vi "Cloud2.vi"() -> ()   [LabVIEW 2017]
uses:
  <vilib>/addons/_JKI.lib/REST Client/classes/REST Client/HTTP Header.ctl
  <vilib>/addons/_JKI.lib/REST Client/classes/REST Client/REST Client.lvclass
panel:
  out "error out 3":errorcluster
  out "error out 2":errorcluster
  out "F-format string":string
  in  "stop":bool
  out "Response body":string
  out "error out":errorcluster
  in  "Default Headers ([JSON])":T1[](array[typedef])=[{"header"="Content-Type", "value"="application/json"}]
  in  "error in (no error)":errorcluster
  in  "Authentication":cluster{"Username":string, "Password":string}
  in  "Base URL":string
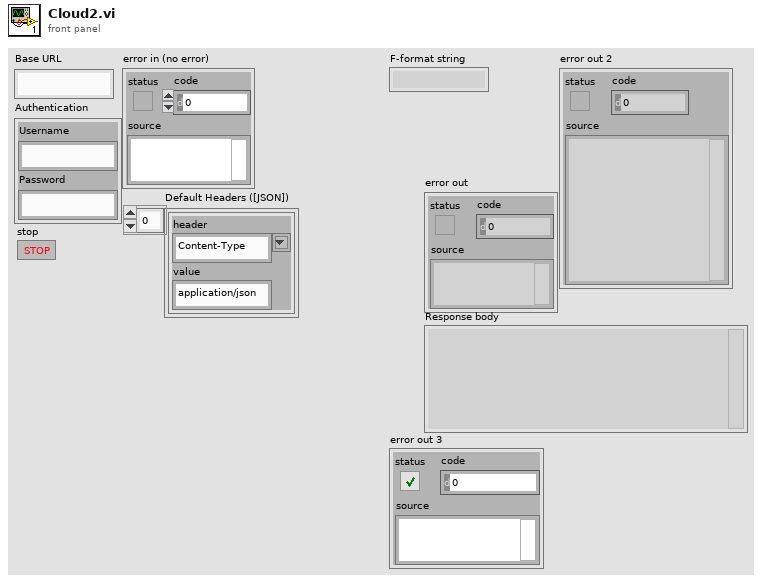
[diagram p1: front panel]
types:
  T1 = typedef "REST Client.lvlib/REST Client.lvclass/HTTP Header.ctl" = cluster{"header":string, "value":string}
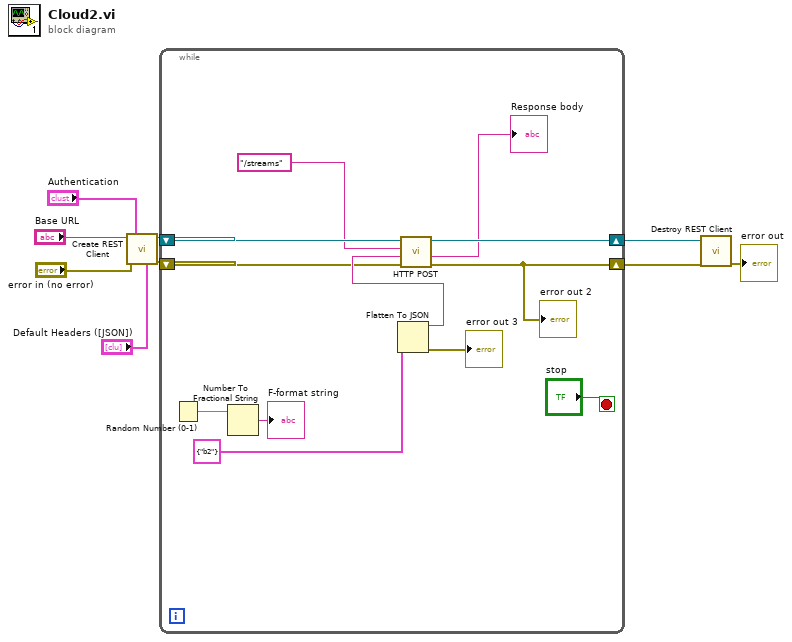
[diagram p0: block diagram]
diagram:
  n1 = call <vilib>:"Create REST Client.vi"("Default Headers ([JSON])"="Default Headers ([JSON])", "error in (no error)"="error in (no error)", "Authentication"="Authentication", "Base URL"="Base URL") -> ("error out"=w3:errorcluster, "REST Client out"=w9:refnum<class "REST Client.lvclass">)  [unwired: 6 in]
  n2 = while {
    shift-right: [w20] -> w8
    shift-left: w9 -> [w21]
    shift-right: [w11] -> w2
    shift-left: w3 -> [w14]
    stop <- "stop" stop-if-true
    n3 = Random Number (0-1)() -> (number: 0 to 1=w16:dbl)
    n4 = Number To Fractional String(number=w16) -> (F-format string=→"F-format string":string)  [unwired: 3 in]
    n5 = Flatten To JSON(anything=cluster{string} {"b2"}) -> (JSON string=w15:string, 11:→"error out 3":errorcluster)  [unwired: 2 in]
    n6 = call-dynamic "HTTP POST.vi"("error in (no error)"=w14, "Request body"=w15, "Path"="/streams", "REST Client in"=w21) -> ("error out"=w11:errorcluster, "Response body"=→"Response body":string, "REST Client out"=w20:refnum<class "REST Client.lvclass">)  [unwired: 2 in, 3 out]
    "error out 2" <- w11
  }
  n7 = call-dynamic "Destroy REST Client.vi"("error in (no error)"=w2, "REST Client in"=w8) -> ("error out"=→"error out":errorcluster)  [unwired: 9 in]
